vi "Write PV_index_simple.vi"(10 "PV_index":i32, 11 "Heater in":refnum<class "Heater.lvclass">) -> (2 "Find":bool, 3 "Heater out":refnum<class "Heater.lvclass">)   [LabVIEW 2019, in "Heating.lvlib" / "Heater.lvclass"]
uses:
  Heater.lvclass
  Heater.lvclass/Heater.ctl
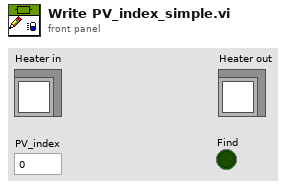
[diagram p1: front panel]
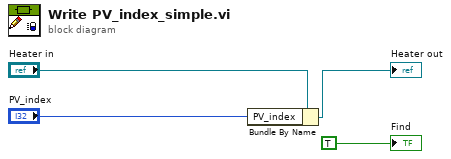
[diagram p0: block diagram]
diagram:
  n1 = Bundle By Name(cluster="Heater in", "PV_index"="PV_index") -> (→"Heater out":refnum<class "Heater.lvclass">)
  "Find" <- TRUE
